vi "Update from Up.vi"(9 "Col":i32, 10 "Row":i32, 11 "Proto in":refnum<class "Proto.lvclass">) -> (3 "Proto out":refnum<class "Proto.lvclass">)   [LabVIEW 2021, in "Proto.lvclass"]
uses:
  Proto.lvclass
  Proto.lvclass/Proto.ctl
  Direction.ctl
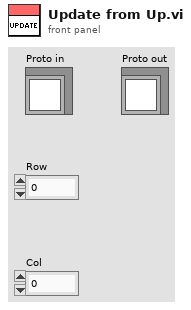
[diagram p1: front panel]
types:
  T1 = typedef "Proto.lvclass/Direction.ctl" = enum16{"Up", "Down", "Right", "Left"}
  T2 = map{cluster{"Row":i32, "Col":i32}, set{cluster{"Heat":i32, "Prev Steps":T1[]}}}
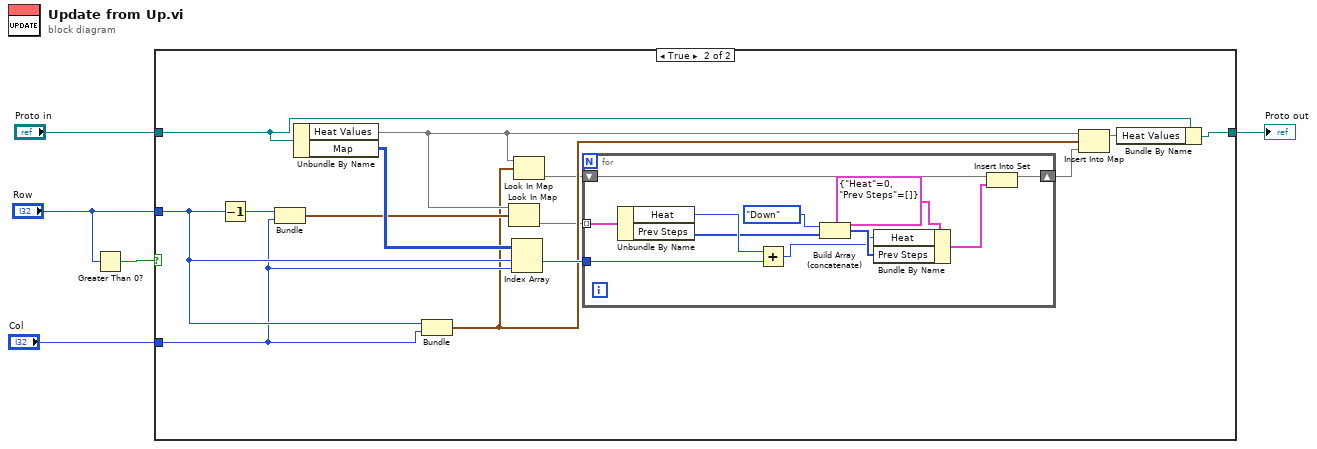
[diagram p0: block diagram]
diagram:
  n1 = Greater Than 0?(x="Row") -> (x > 0?=w1:bool)
  n2 = case shown="True" w1 {
    tunnel: [w6 w18] -> w5
    tunnel: "Proto in" -> [w6 w17]
    tunnel: "Row" -> [_ w14]
    tunnel: "Col" -> [_ w13]
    frame False {
    }
    frame True {
      n3 = Decrement(x=w14) -> (x-1=w12:i32)
      n4 = Bundle(w12, "Col"=w13) -> (w16:cluster{i32, "Col":i32})  [unwired: 1 in]
      n5 = Unbundle By Name(w17) -> ("Heat Values"=w10:T2, "Map"=w20:i32[][])
      n6 = Bundle("Row"=w14, "Col"=w13) -> (w9:cluster{"Row":i32, "Col":i32})  [unwired: 1 in]
      n7 = Look In Map(map=w10, key=w16) -> (value=w8:set{cluster{"Heat":i32, "Prev Steps":T1[]}})  [unwired: 1 in, 1 out]
      n8 = Index Array(array=w20, index (row)=w14, index (col)=w13) -> (element=w15:i32)
      n9 = Look In Map(map=w10, key=w9) -> (value=w7:set{cluster{"Heat":i32, "Prev Steps":T1[]}})  [unwired: 1 in, 1 out]
      n10 = for {
        tunnel: w15 -> [w30]
        shift-right: [w23] -> w11
        shift-left: w7 -> [w24]
        tunnel: w8 -> [w25] mode=indexing
        n11 = Unbundle By Name(w25) -> ("Heat"=w31:i32, "Prev Steps"=w29:T1[])
        n12 = Add(x=w31, y=w30) -> (x+y=w26:i32)
        n13 = Build Array (concatenate)(Direction."Down" ("Dir"), w29) -> (w27:T1[])
        n14 = Bundle By Name(cluster=cluster{"Heat":i32, "Prev Steps":T1[]} {"Heat"=0, "Prev Steps"=[]} ("element"), "Heat"=w26, "Prev Steps"=w27) -> (w21:cluster{"Heat":i32, "Prev Steps":T1[]})
        n15 = Insert Into Set(10:w21, 11:w24) -> (3:w23:set{cluster{"Heat":i32, "Prev Steps":T1[]}})  [unwired: 1 out]
      }
      n16 = Insert Into Map(map in=w10, key=w9, value=w11) -> (map out=w19:T2)  [unwired: 2 out]
      n17 = Bundle By Name(cluster=w17, "Heat Values"=w19) -> (w18:refnum<class "Proto.lvclass">)
    }
  }
  "Proto out" <- w5
